vi "Read DVR.vi"(8 "error in (no error)":errorcluster, 11 "Data Subject in":refnum<class "Data Subject.lvclass">) -> (0 "error out":errorcluster, 2 "DVR":refnum<data-value>, 3 "Data Subject out":refnum<class "Data Subject.lvclass">)   [LabVIEW 2018, in "Data Subject.lvclass"]
uses:
  Data Subject.lvclass
  Data/Data.lvclass
  Data Subject.lvclass/Data Subject.ctl
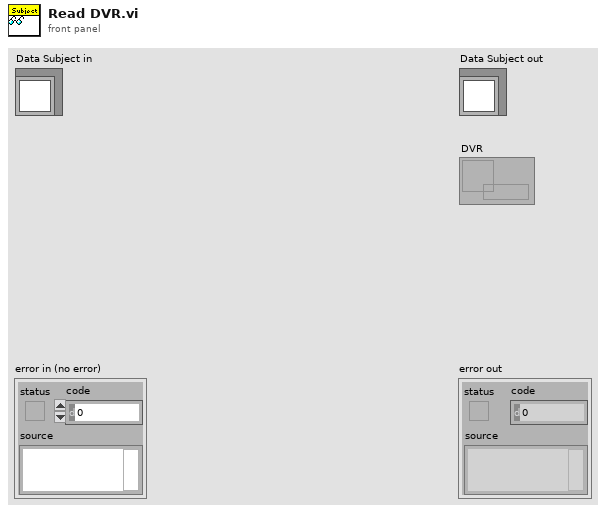
[diagram p1: front panel]
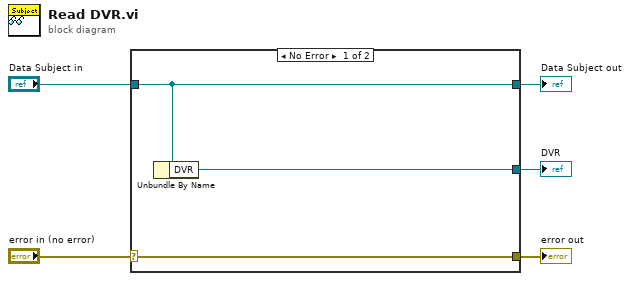
[diagram p0: block diagram]
diagram:
  n1 = case shown="No Error" "error in (no error)" {
    selector: "error in (no error)" -> [w8 w9]
    tunnel: [w8 w9] -> w4
    tunnel: [w7 w10] -> w2
    tunnel: "Data Subject in" -> [w7 w10]
    tunnel: [w6 _] -> w1
    frame No Error {
      n2 = Unbundle By Name(w7) -> ("DVR"=w6:refnum<data-value>)
    }
    frame Error {
    }
  }
  "error out" <- w4
  "Data Subject out" <- w2
  "DVR" <- w1
